vi "Self-Test.vi"(8 "error in (no error)":errorcluster, 11 "VISA resource name":refnum<visa-resource-name>) -> (0 "error out":errorcluster, 1 "Self-Test Result Message":string, 2 "Self-Test Result Code":i32, 3 "VISA resource name out":refnum<visa-resource-name>)   [LabVIEW 2009, in "Tektronix AFG 3000 Series.lvlib"]
doc: "Runs the instrument's self test routine and returns the test results."
uses:
  Tektronix AFG 3000 Series.lvlib
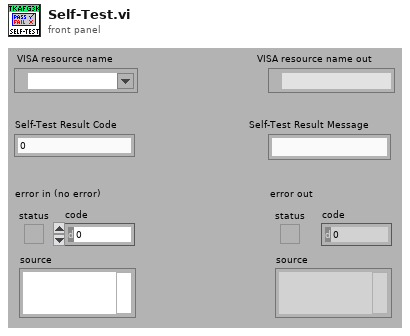
[diagram p1: front panel]
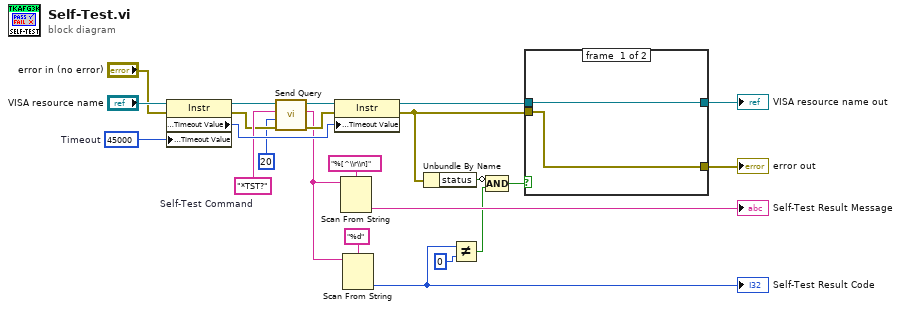
[diagram p0: block diagram]
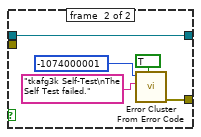
[diagram p2: hidden frame]
diagram:
  w19 = u32 45000  # Timeout
  w9 = "*TST?"  # Self-Test Command
  n1 = property class="Instr"(reference="VISA resource name", error in="error in (no error)", "General Settings:Timeout Value"=w19) -> (reference out=w8:refnum<visa-resource-name>, error out=w7:errorcluster, "General Settings:Timeout Value"=w18:u32)
  n2 = call "Send Query.vi"("error in (no error)"=w7, "byte count (1024)"=u32 20 ("byte count (20)"), "write buffer"=w9, "VISA resource name"=w8) -> ("error out"=w4:errorcluster, "read buffer"=w3:string, "VISA resource name out"=w5:refnum<visa-resource-name>)  [unwired: 5 out]
  n3 = property class="Instr"(reference=w5, error in=w4, "General Settings:Timeout Value"=w18) -> (reference out=w17:refnum<visa-resource-name>, error out=w16:errorcluster)
  n4 = Scan From String(format string="%[^\\r\\n]" ("Format String"), input string=w3) -> (output 1=→"Self-Test Result Message":string)  [unwired: 2 in, 4 out]
  n5 = Scan From String(format string="%d", input string=w3) -> (output 1=w12:i32)  [unwired: 2 in, 4 out]
  "Self-Test Result Code" <- w12
  n6 = Unbundle By Name(w16) -> ("status"=w14:bool)
  n7 = Not Equal?(x=w12, y=0) -> (x != y?=w15:bool)
  n8 = Compound Arithmetic op=AND(invert w14, w15) -> (w13:bool)
  n9 = case shown="True" w13 {
    tunnel: w17 -> [w25 w30]
    tunnel: w16 -> [w24 _]
    tunnel: [w24 w26] -> w2
    tunnel: [w25 w30] -> w1
    frame #0 {
    }
    frame #1 {
      n10 = call <vilib>:"Error Cluster From Error Code.vi"("show call chain? (False)"=TRUE ("Status"), "error message (\"\")"="tkafg3k Self-Test\nThe Self Test failed." ("Source (VI Name)"), "error code (0)"=-1074000001 ("Code")) -> ("error out"=w26:errorcluster)  [unwired: 1 in, 5 out]
    }
  }
  "VISA resource name out" <- w1
  "error out" <- w2
